vi "Confocal_0919_withZstep.vi"() -> ()   [LabVIEW 2017]
uses:
  <vilib>/Math Plots/2D Math Plots/XY Plot Matrix/XY Plot Matrix XCtrl/XY Plot Matrix.xctl
  Public/Documents/SIToolkit/LabVIEW/ExamplesXX_4_3_1_4/Spectroscopy Applications/GlobalCamOpen.vi
  Public/Documents/SIToolkit/LabVIEW/ExamplesXX_4_3_1_4/Spectroscopy Applications/GlobalInitializeFlag.vi
  Desktop/GlobalTimingMode-edit.vi
  Public/Documents/SIToolkit/LabVIEW/ExamplesXX_4_3_1_4/Spectroscopy Applications/GlobalFramesToStr.vi
  Public/Documents/SIToolkit/LabVIEW/ExamplesXX_4_3_1_4/Spectroscopy Applications/GlobalAcquireFocusFlag.vi
  Public/Documents/SIToolkit/LabVIEW/ExamplesXX_4_3_1_4/Spectroscopy Applications/GlobalExposure.vi
  <vilib>/Math Plots/2D Math Plots/XY Plot Matrix/XY Plot Matrix Datatype/XY Plot Matrix Datatype.lvclass
panel:
  out "Position 6":dbl[](array[numeric]) format="%.6f"
  out "Position 7":dbl[](array[numeric]) format="%.6f"
  out "Position 4":dbl[](array[numeric]) format="%.6f"
  in  "error PI Stage":errorcluster
  out "error out 2":errorcluster
  in  "Tab Control":T1(tab)
  in  "Focus/Acquire Mode":u32=1 min=1 max=5 step=1
  in  "Number of Frames to store":u32=1 min=1 step=1
  in  "Timing Mode":u32(ring)=1 items=["N/A", "Free Run/Timed", "Trigger First (PM only)", "Ext Sync/Strobed ", "Variable Exp (PM only)", "Flash Mode (PM only)"]
  out "Pixel Time":i32
  out "Bit Depth":i32
  out "ReadOut port":i32
  out "ADC Speed":i32
  in  "Set Experiment \nParameters, Initialize \nCamera/Controller":bool
  out "Read Temp.":dbl format="%.2f"
  in  "Set Temp.":dbl format="%.2f"
  in  "Exposure 2":dbl=0.2 format="%.2f"
  out "Controller Initialized":bool
  in  "error in":errorcluster
  out "error out":errorcluster
  in  "Power":dbl=10.0
  in  "Frequency":dbl=2810.0
  in  "Release Camera":bool
  out "Camera Opened":bool
  out "COM Error":bool
  in  "Serial Port":refnum<visa-resource-name>="COM3"
  in  "Number of Steps Left (must be even)":dbl=5.0 format="%#_13g"
  in  "OK Button 5":bool
  in  "Step Size (microns)":dbl[](array[numeric])=[0.01]
  out "XY Plot Matrix":refnum<class "XY Plot Matrix Datatype.lvclass">[](xcontrol)
  in  "Number of Steps Down":dbl=5.0 format="%#_13g"
  out "Position":dbl[](array[numeric]) format="%.6f"
  out "Position 3":dbl[](array[numeric]) format="%.6f"
  in  "stop 2":bool
  out "Position 2":dbl[](array[numeric]) format="%.6f"
  out "loop iteration":i32
  in  "Step Size (microns) Z":dbl[](array[numeric])=[0.01]
  out "Execution Time (ms)":u32
  in  "?":bool
  out "Position 5":dbl[](array[numeric]) format="%.6f"
  in  "Step Size (microns) Y":dbl[](array[numeric])=[0.01]
  in  "Step Size (microns) X":dbl[](array[numeric])=[0.01]
  out "Position 8":dbl[](array[numeric]) format="%.6f"
  in  "?":bool
  out "Acquire Graph":sgl[](graph)
  out "Collecting Data":bool
  in  "Full File Name for Acqure":path
  in  "OK Button":bool
  # "The following are read \nfrom camera after setting\nvalues to left.\n-1 value means item is not \nsupported by camera."
  # "Stage position on connection."
  # "Be sure to put in a full file name below before starting."
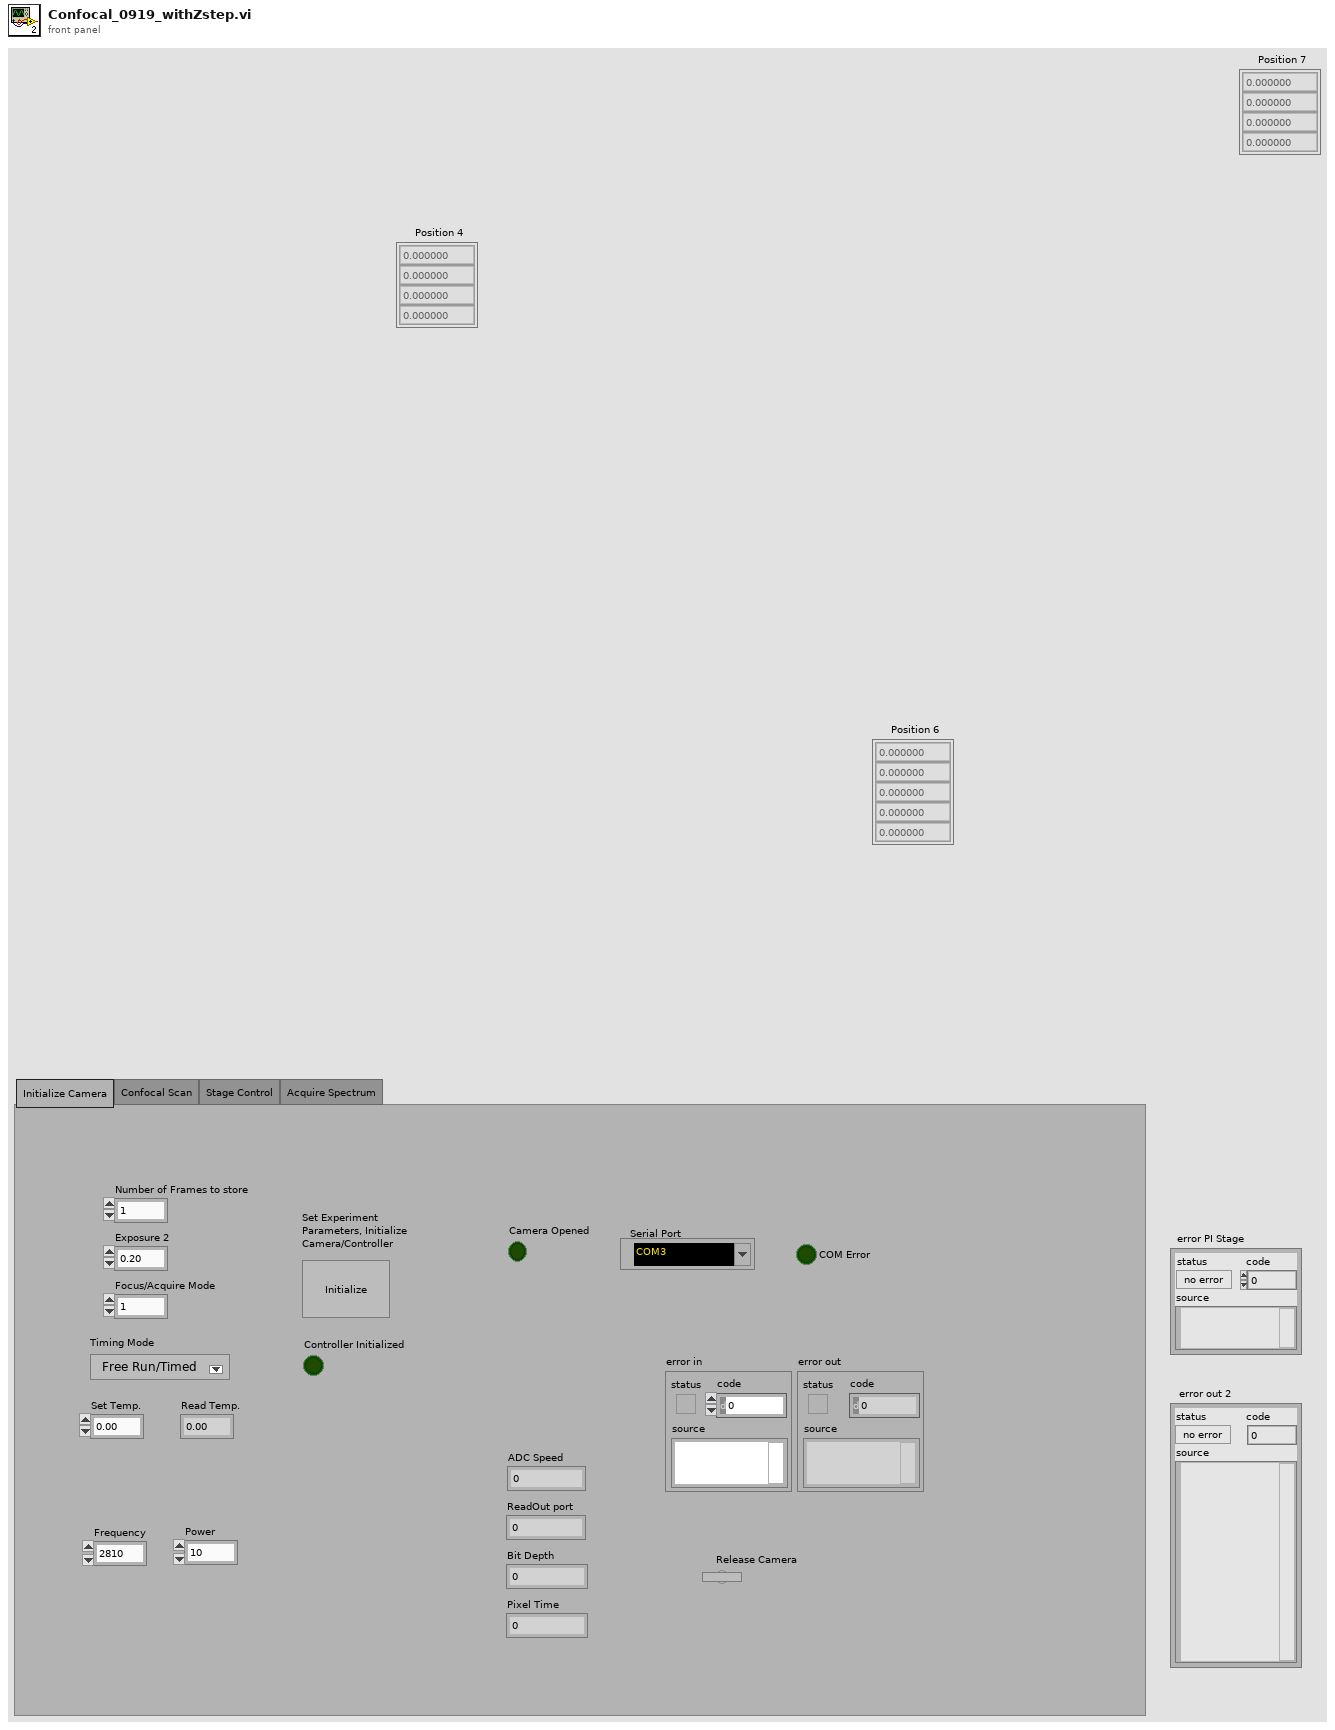
[diagram p1: front panel]
types:
  T1 = enum32{"Initialize Camera", "Confocal Scan", "Stage Control", "Acquire Spectrum"}
  T2 = cluster{"X start":u32, "X end":u32, "X Binning/Grouping":u32, "Y start":u32, "Y end":u32, "Y Binning/Grouping":u32}
  T3 = cluster{"Camera Handle":u32, "Pulser Handle":u32, "File Handle":u32, "Display Handle":u32, "Image Handle":u32}
  T4 = cluster{"Host address/name":string, "Port":i32, "Board":i32, "TCP/IP Search?":bool}
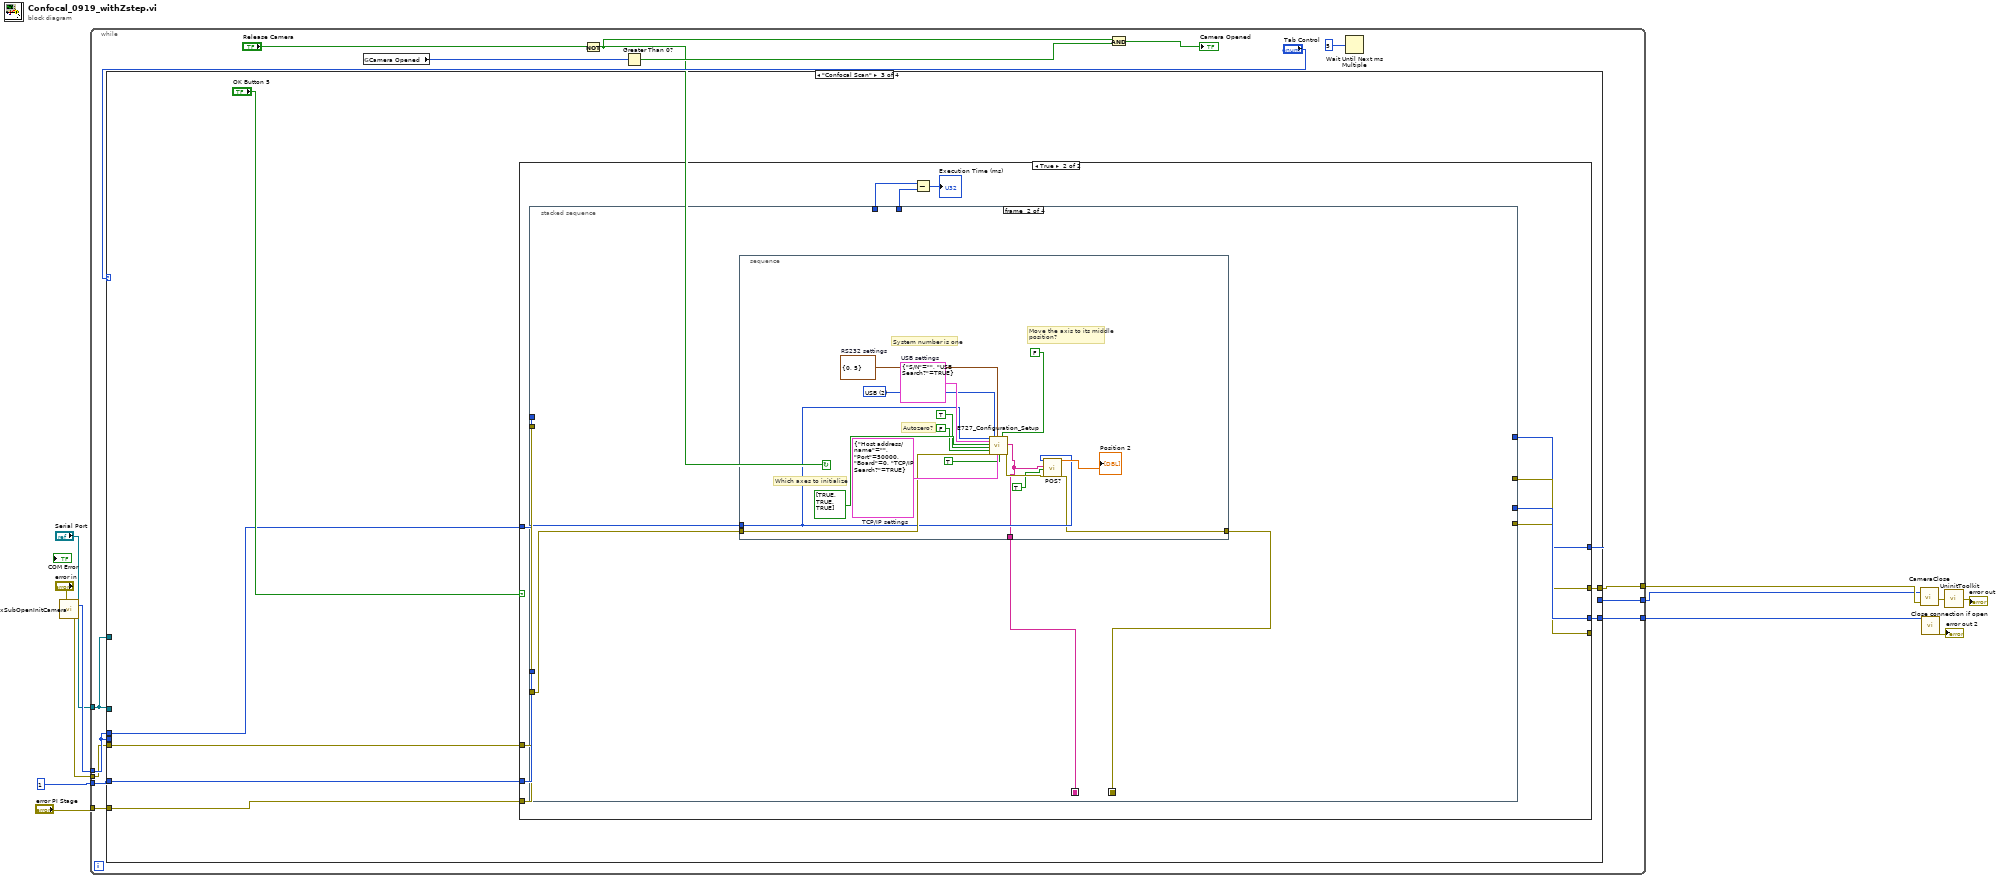
[diagram p0: block diagram]
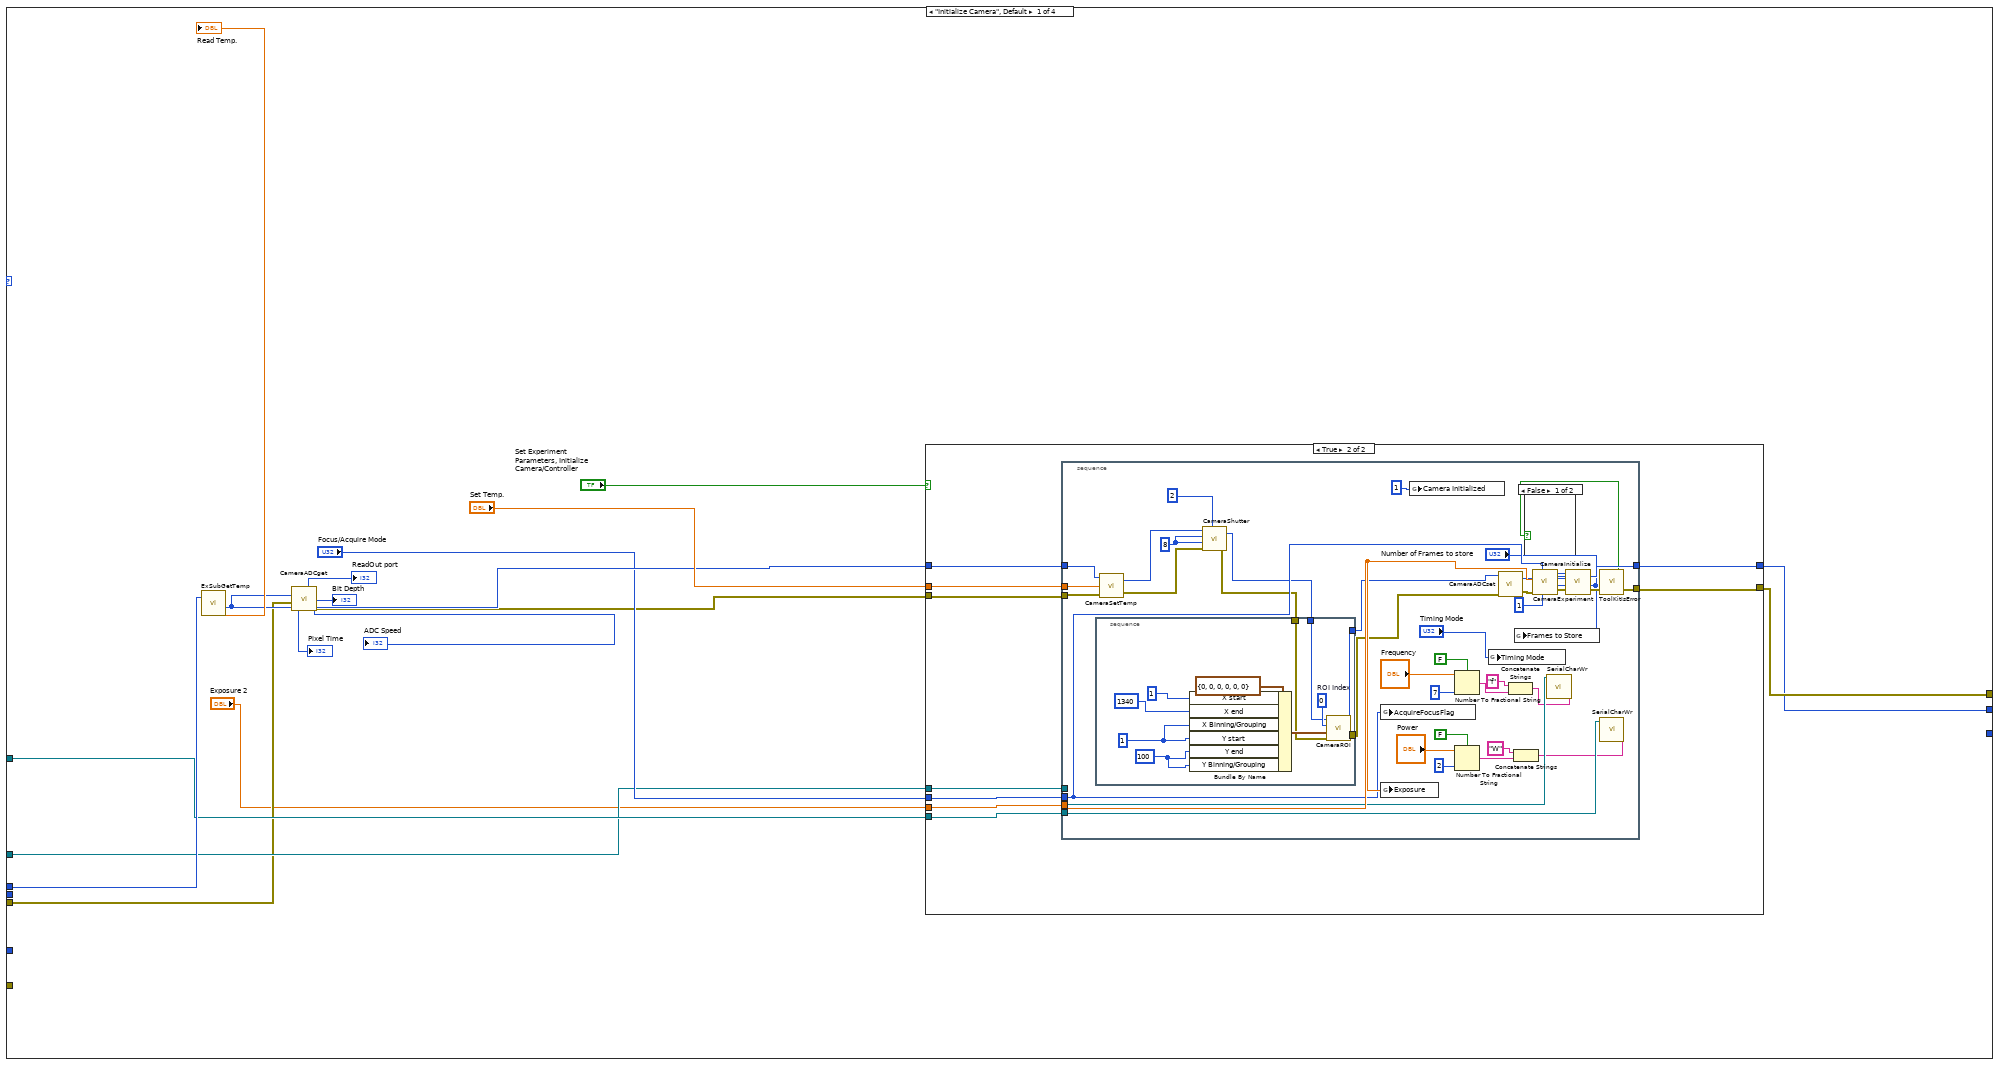
[diagram p2: hidden frame]
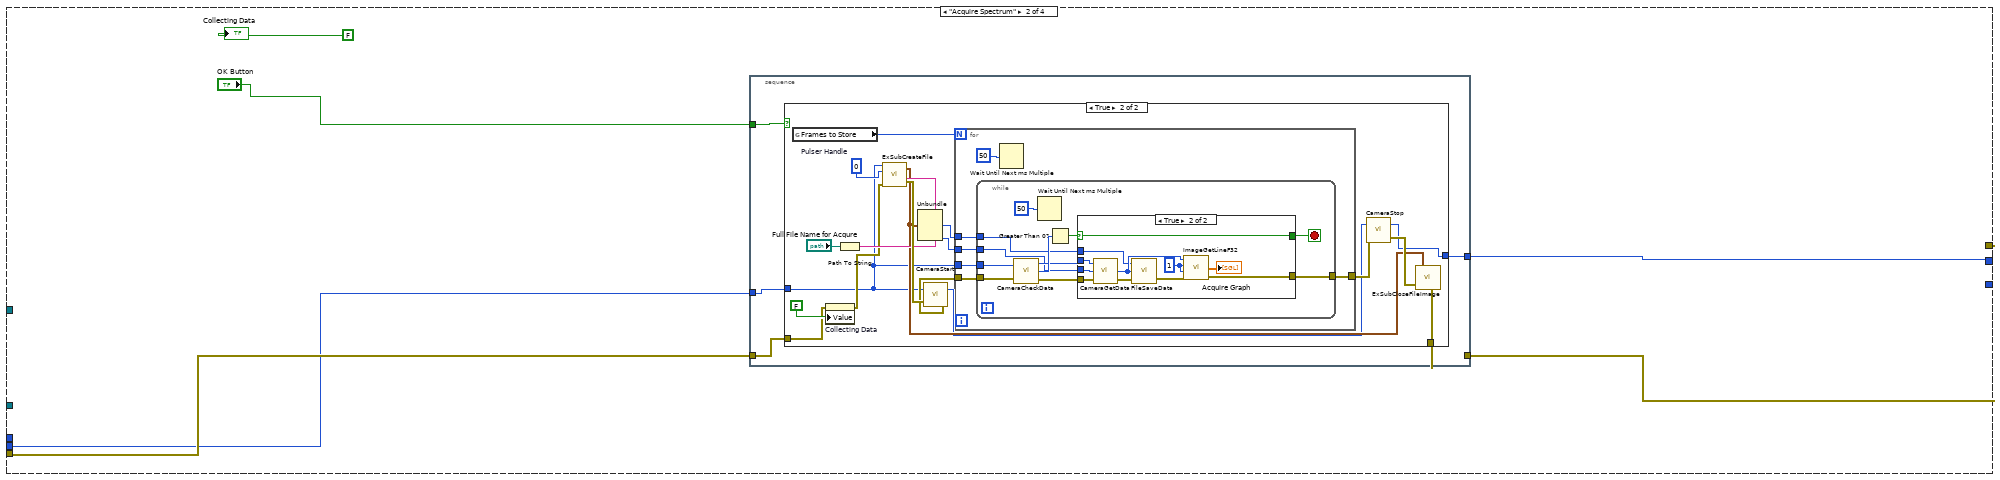
[diagram p5: hidden frame]
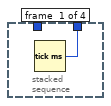
[diagram p9: hidden frame]
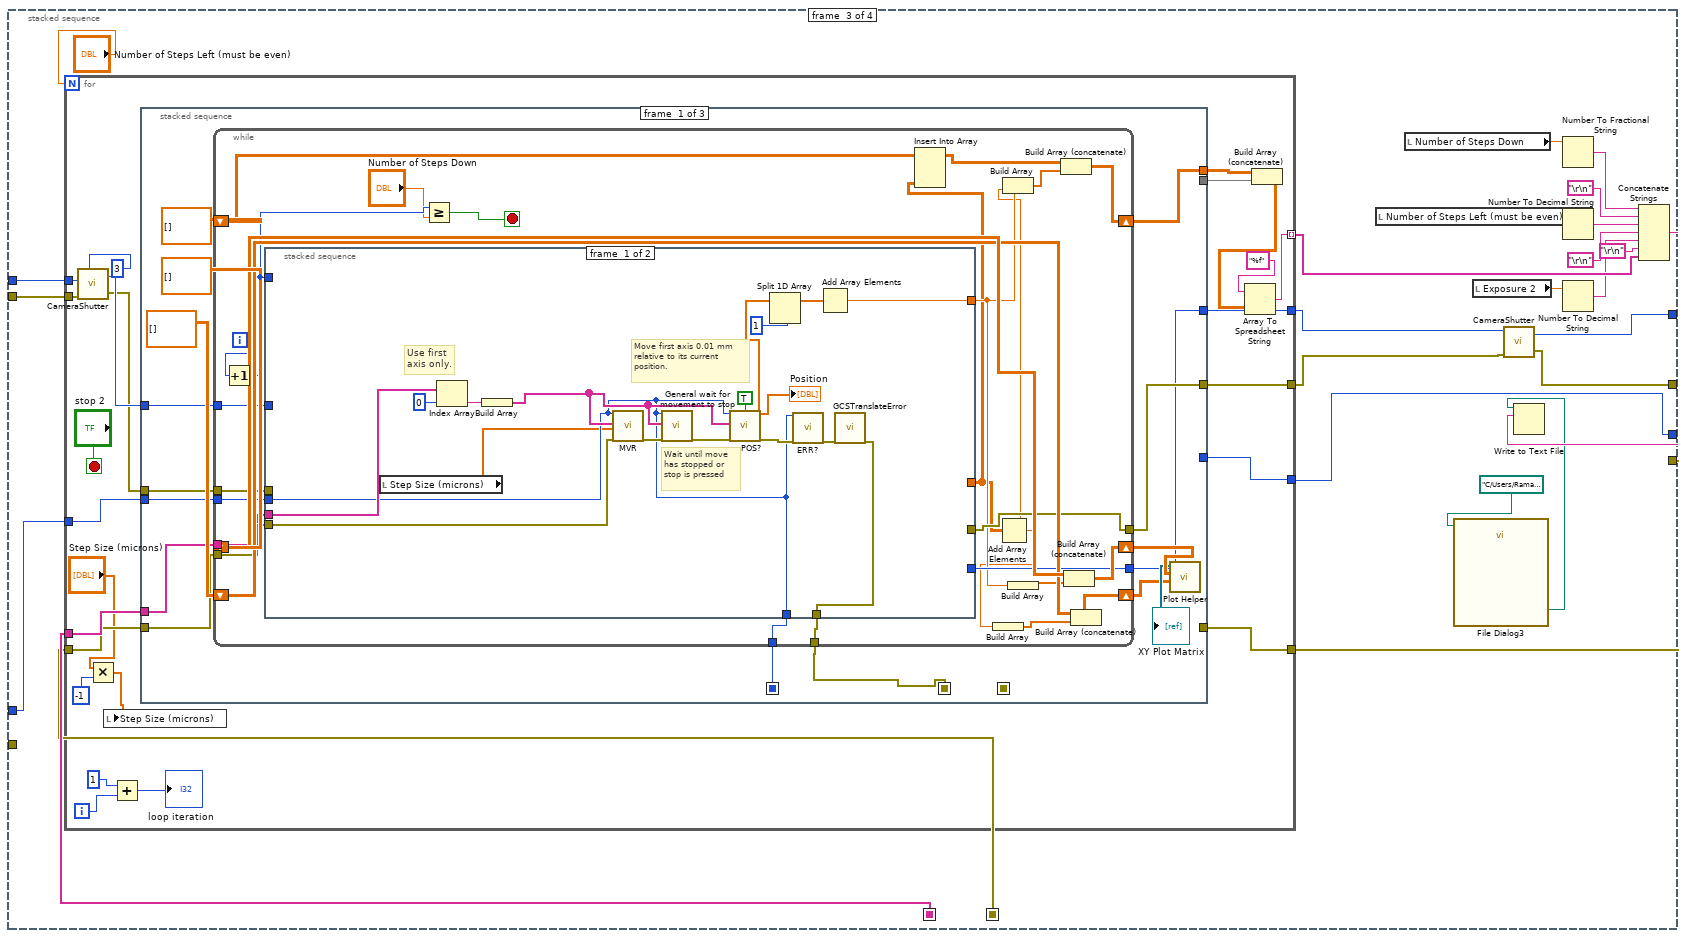
[diagram p10: hidden frame]
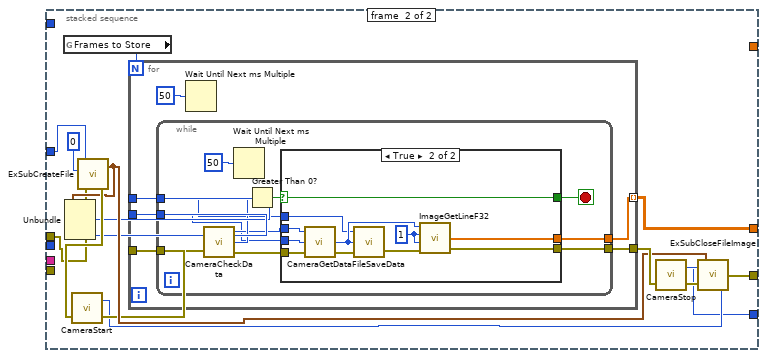
[diagram p11: hidden frame]
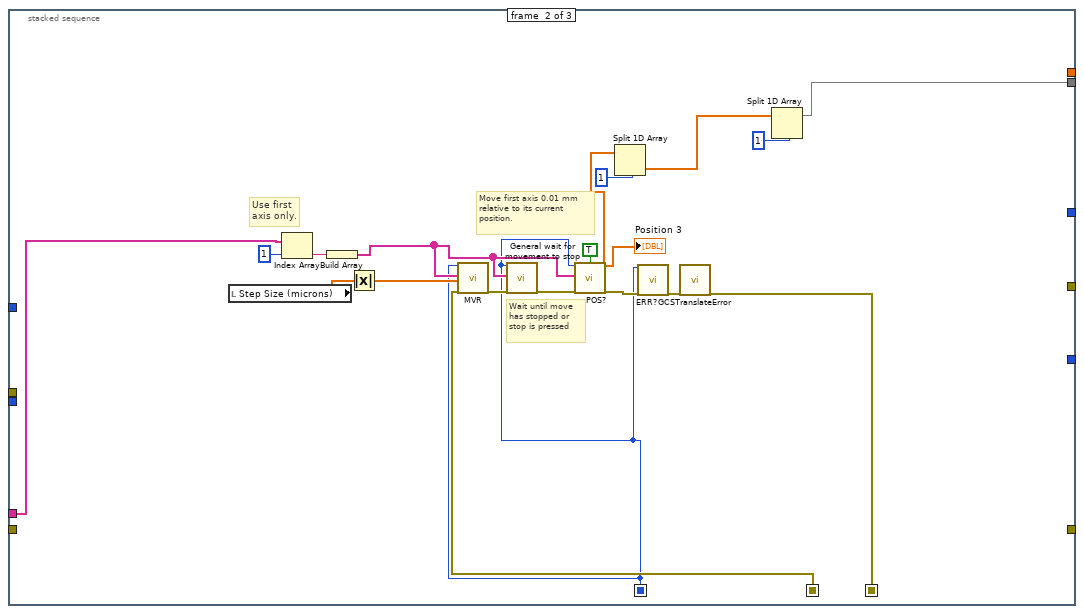
[diagram p13: hidden frame]
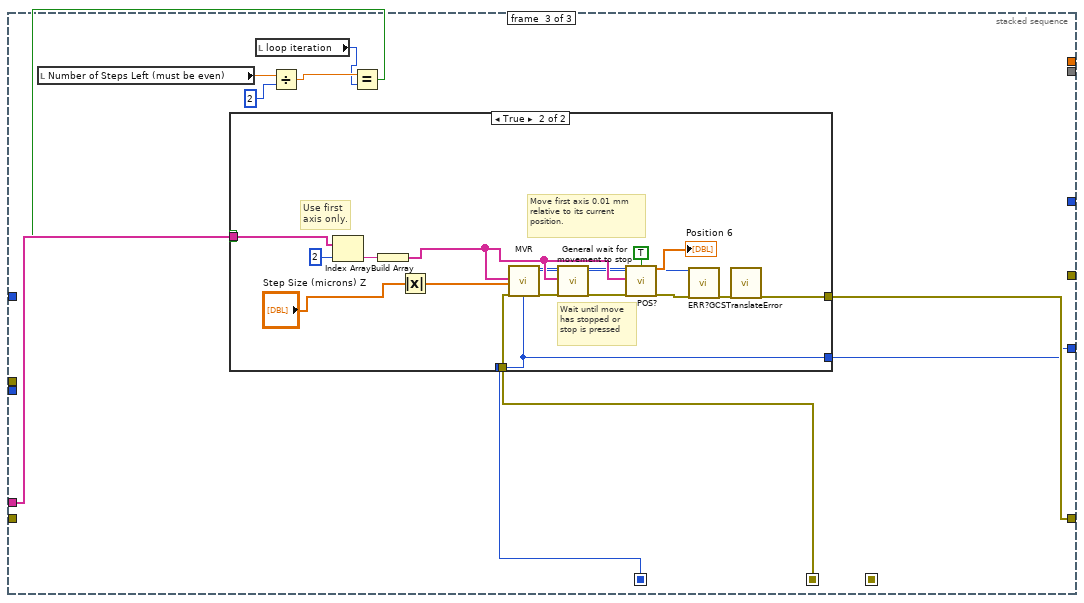
[diagram p14: hidden frame]
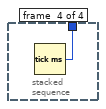
[diagram p16: hidden frame]
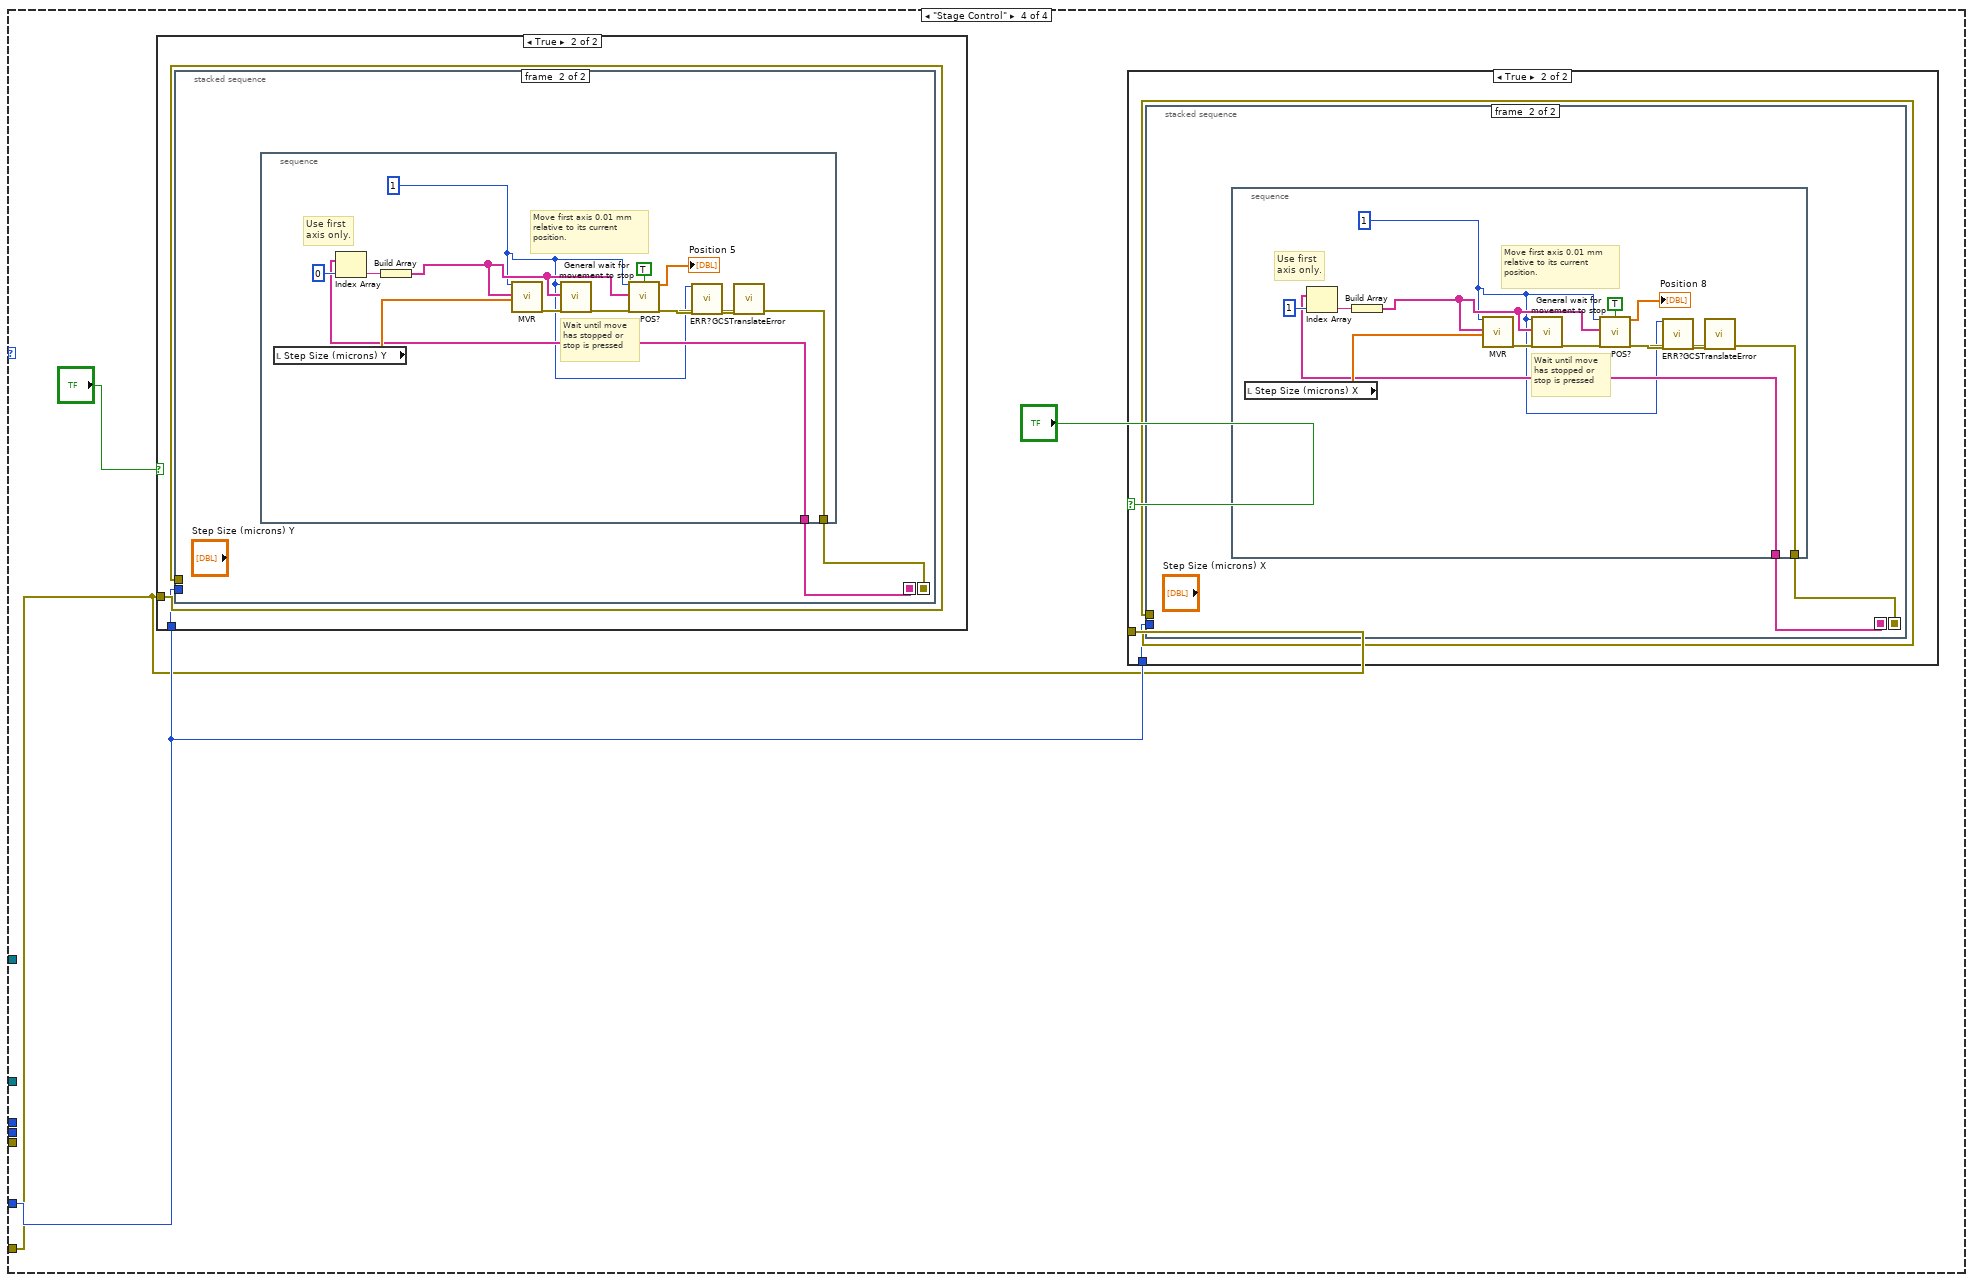
[diagram p17: hidden frame]
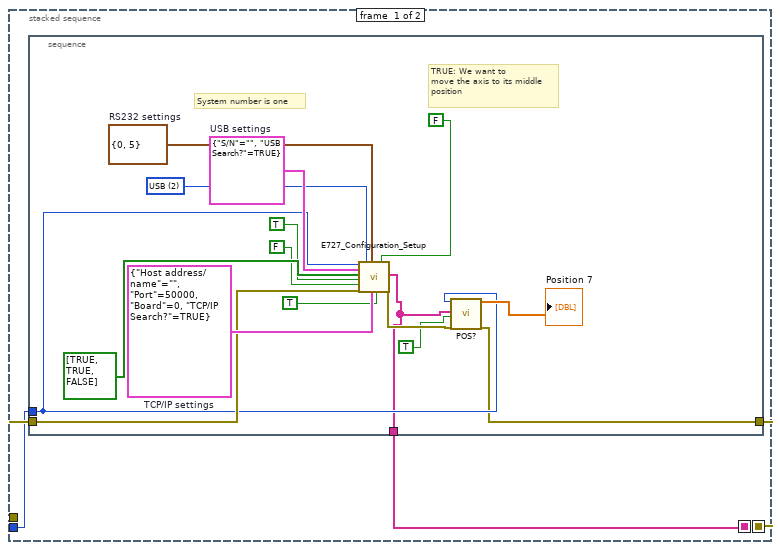
[diagram p19: hidden frame]
diagram:
  n1 = call "ExSubOpenInitCamera.vi"("error in (no error)"="error in") -> ("Camera Handle"=w11:u32, "error out"=w9:errorcluster)
  n2 = while {
    tunnel: w11 -> [w20]
    tunnel: "Serial Port" -> [w21]
    tunnel: w9 -> [w19]
    tunnel: [w18] -> w8
    tunnel: [w16] -> w5
    tunnel: "error PI Stage" -> [w15]
    tunnel: 1 -> [w13]
    tunnel: [w14] -> w1
    stop <- w17 continue-if-true
    n3 = case shown="\"Confocal Scan\"" "Tab Control" {
      tunnel: w20 -> [w36 _ w169 _]
      tunnel: w21 -> [w35 _ _ _]
      tunnel: w21 -> [w34 _ _ _]
      tunnel: w20 -> [_ w111 _ _]
      tunnel: w19 -> [w33 w112 w170 _]
      tunnel: [w28 w108 w171 _] -> w16
      tunnel: [w30 w109 w172 _] -> w18
      tunnel: w15 -> [_ _ w174 w409]
      tunnel: w13 -> [_ _ w176 w410]
      tunnel: [_ _ w175 _] -> w14
      frame "Initialize Camera", Default {
        n4 = call "ExSubGetTemp.vi"("Camera Handle"=w36) -> ("Camera Handle"=w41:u32, "Temperature Real"=→"Read Temp.":dbl)  [unwired: 1 in, 1 out]
        n5 = call <userlib>:"CameraADCget.vi"("Camera handle"=w41, "error in (no error)"=w33) -> ("Bit Depth"=→"Bit Depth":i32, "Pixel Time"=→"Pixel Time":i32, "Readout Port"=→"ReadOut port":i32, "ADC Speed"=→"ADC Speed":i32, "error out"=w32:errorcluster)  [unwired: 3 out]
        n6 = case shown="True" "Set Experiment \nParameters, Initialize \nCamera/Controller" {
          tunnel: "Exposure 2" -> [_ w55]
          tunnel: "Set Temp." -> [_ w56]
          tunnel: w41 -> [w48 w57]
          tunnel: [w48 w54] -> w28
          tunnel: "Focus/Acquire Mode" -> [_ w53]
          tunnel: w35 -> [_ w52]
          tunnel: w34 -> [_ w51]
          tunnel: w32 -> [w47 w50]
          tunnel: [w47 w49] -> w30
          frame False {
          }
          frame True {
            n7 = stacked-sequence {
              tunnel: w57 -> [w96]
              tunnel: w56 -> [w95]
              tunnel: w55 -> [w94]
              tunnel: [w93] -> w54
              tunnel: w53 -> [w92]
              tunnel: w52 -> [w91]
              tunnel: w51 -> [w90]
              tunnel: w50 -> [w89]
              tunnel: [w88] -> w49
              frame #0 {
                w58 = 8
                n8 = call <userlib>:"CameraSetTemp.vi"("error in (no error)"=w89, "Temperature"=w95, "Camera Handle"=w96) -> ("error out"=w61:errorcluster, "Camera Handle"=w63:u32)
                n9 = call <userlib>:"CameraShutter.vi"("Camera Handle"=w63, "Shutter Comp Time: Pre Open"=w58, "Shutter Comp Time: Post Open"=w58, "error in"=w61, "Shutter State"=2) -> ("Camera Handle"=w62:u32, "error out"=w60:errorcluster)
                n10 = stacked-sequence {
                  tunnel: [w104] -> w65
                  tunnel: w62 -> [w101]
                  tunnel: w60 -> [w100]
                  tunnel: [w99] -> w64
                  frame #0 {
                    w103 = 100
                    w97 = 1
                    w106 = u32 0  # ROI Index
                    n11 = Bundle By Name(cluster=T2 {"X start"=0, "X end"=0, "X Binning/Grouping"=0, "Y start"=0, "Y end"=0, "Y Binning/Grouping"=0} ("ROI Params"), "X start"=1, "X end"=1340, "X Binning/Grouping"=w97, "Y start"=w97, "Y end"=w103, "Y Binning/Grouping"=w103) -> (w107:T2)
                    n12 = call <userlib>:"CameraROI.vi"("error in"=w100, "ROI Params"=w107, "ROI Index"=w106, "Camera Handle"=w101) -> ("error out"=w99:errorcluster, "Camera Handle"=w104:u32)
                  }
                }
                n13 = global write "GlobalAcquireFocusFlag.vi" "AcquireFocusFlag"(w92) -> ()
                n14 = global write "GlobalExposure.vi" "Exposure"(w94) -> ()
                n15 = global write "GlobalInitializeFlag.vi" "Camera Initialized"(1) -> ()
                n16 = Number To Fractional String(use system decimal point (T)=FALSE, number="Frequency", precision (6)=7) -> (F-format string=w67:string)  [unwired: 1 in]
                n17 = Number To Fractional String(use system decimal point (T)=FALSE, number="Power", precision (6)=2) -> (F-format string=w75:string)  [unwired: 1 in]
                n18 = global write "GlobalTimingMode-edit.vi" "Timing Mode"("Timing Mode") -> ()
                n19 = call <userlib>:"CameraADCset.vi"("error in (no error)"=w64, "Camera Handle"=w65) -> ("error out"=w84:errorcluster, "Camera Handle"=w83:u32)  [unwired: 4 in]
                n20 = Concatenate Strings("f", w67) -> (w73:string)
                n21 = Concatenate Strings("W", w75) -> (w76:string)
                n22 = global write "GlobalFramesToStr.vi" "Frames to Store"("Number of Frames to store") -> ()
                n23 = call <userlib>:"CameraExperiment.vi"("Number of Accumulations"=1, "Acquire / Focus Flag"=w92, "error in"=w84, "Number of Images"="Number of Frames to store", "Exposure (sec)"=w94, "Camera Handle"=w83) -> ("error out"=w82:errorcluster, "Camera Handle"=w81:u32)
                n24 = call "SerialCharWr.vi"("VISA resource name"=w90, "write buffer"=w73) -> ()  [unwired: 6 in, 3 out]
                n25 = call <userlib>:"CameraInitialize.vi"("error in"=w82, "Camera Handle"=w81) -> ("error out"=w79:errorcluster, "Camera Handle"=w93:u32)
                n26 = call <userlib>:"ToolKitIsError.vi"("error in"=w79) -> ("error out"=w88:errorcluster, "Error Flag"=w80:bool)  [unwired: 1 in]
                n27 = case shown="False" w80 {
                  frame False {
                  }
                  frame True {
                  }
                }
                n28 = call "SerialCharWr.vi"("VISA resource name"=w91, "write buffer"=w76) -> ()  [unwired: 6 in, 3 out]
              }
            }
          }
        }
        n29 = global read "GlobalInitializeFlag.vi" "Camera Initialized"() -> (w44:u32)
        n30 = Greater Than 0?(x=w44) -> (x > 0?=→"Controller Initialized":bool)
      }
      frame "Acquire Spectrum" {
        n31 = stacked-sequence {
          tunnel: [w115] -> w109
          tunnel: [w116] -> w108
          tunnel: w112 -> [w118]
          tunnel: "OK Button" -> [w117]
          tunnel: w111 -> [w114]
          frame #0 {
            n32 = case shown="True" w117 {
              tunnel: [w119 w131] -> w116
              tunnel: [w120 w123] -> w115
              tunnel: w118 -> [w120 w122]
              tunnel: w114 -> [w119 w121]
              frame False {
              }
              frame True {
                w125 = u32 0  # Pulser Handle
                n33 = global read "GlobalFramesToStr.vi" "Frames to Store"() -> (w134:u32)
                n34 = property on="Collecting Data" class="Bool (strict)"(error in=w122, "Value"=FALSE) -> (error out=w133:errorcluster)  [unwired: 1 in, 1 out]
                n35 = Path To String(path="Full File Name for Acqure") -> (string=w136:string)
                n36 = call "ExSubCreateFile.vi"("error in (no error)"=w133, "File and Display Name"=w136, "Pulser Handle"=w125, "Camera Handle"=w121) -> ("error out"=w138:errorcluster, "Handles Out"=w129:T3)
                n37 = Unbundle(w129) -> ("File Handle"=w124:u32, "Image Handle"=w127:u32)  [unwired: 3 out]
                n38 = call <userlib>:"CameraStart.vi"("error in"=w138, "Camera Handle"=w121) -> ("error out"=w128:errorcluster, "Camera Handle"=w126:u32)
                n39 = for {
                  N: w134 -> [_]
                  tunnel: w121 -> [w143]
                  tunnel: w128 -> [w142]
                  tunnel: [w141] -> w130
                  tunnel: w124 -> [w140]
                  tunnel: w127 -> [w139]
                  n40 = while {
                    tunnel: [w150] -> w141
                    tunnel: w143 -> [w148]
                    tunnel: w142 -> [w147]
                    tunnel: w140 -> [w146]
                    tunnel: w139 -> [w145]
                    stop <- w151 stop-if-true
                    n41 = call <userlib>:"CameraCheckData.vi"("Camera Handle"=w148, "error in"=w147) -> ("Camera Handle"=w153:u32, "Number Of Frames Available"=w155:i32, "error out"=w152:errorcluster)
                    n42 = Wait Until Next ms Multiple(millisecond multiple=u32 50) -> ()  [unwired: 1 out]
                    n43 = Greater Than 0?(x=w155) -> (x > 0?=w154:bool)
                    n44 = case shown="True" w154 {
                      selector: w154 -> [w156 w166]
                      tunnel: w153 -> [_ w168]
                      tunnel: w152 -> [w157 w167]
                      tunnel: [w156 w166] -> w151
                      tunnel: [w157 w161] -> w150
                      tunnel: w146 -> [_ w159]
                      tunnel: w145 -> [_ w158]
                      frame False {
                      }
                      frame True {
                        w162 = 1
                        n45 = call <userlib>:"CameraGetData.vi"("error in"=w167, "Image/Data Handle"=w158, "Camera Handle"=w168) -> ("error out"=w165:errorcluster, "Image/Data Handle"=w163:u32)  [unwired: 1 out]
                        n46 = call <userlib>:"FileSaveData.vi"("error in"=w165, "Image Handle"=w163, "File Handle"=w159) -> ("error out"=w164:errorcluster)  [unwired: 1 out]
                        n47 = call <userlib>:"ImageGetLineF32.vi"("error in"=w164, "Z Position"=w162, "Y Position"=w162, "Data Handle"=w163) -> ("error out"=w161:errorcluster, "Array F32"=→"Acquire Graph":sgl[])  [unwired: 1 out]
                      }
                    }
                  }
                  n48 = Wait Until Next ms Multiple(millisecond multiple=u32 50) -> ()  [unwired: 1 out]
                }
                n49 = call <userlib>:"CameraStop.vi"("error in"=w130, "Camera Handle"=w126) -> ("error out"=w135:errorcluster, "Camera Handle"=w131:u32)
                n50 = call "ExSubCloseFileImage.vi"("error in (no error)"=w135, "Handles In"=w129) -> ("error out"=w123:errorcluster)
              }
            }
          }
        }
        "Collecting Data" <- FALSE
      }
      frame "Confocal Scan" {
        n51 = case shown="True" "OK Button 5" {
          tunnel: w176 -> [_ w187]
          tunnel: [_ w186] -> w175
          tunnel: [_ w185] -> _
          tunnel: w174 -> [_ w184]
          tunnel: [_ w183] -> w172
          tunnel: [_ w182] -> w171
          tunnel: w170 -> [_ w181]
          tunnel: w169 -> [_ w180]
          frame False {
          }
          frame True {
            n52 = stacked-sequence {
              seq-local: [_ w190 _ _] -> [_ _ w230 _]
              seq-local: [_ w189 _ _] -> [_ _ w229 _]
              tunnel: w187 -> [_ w191 w233 _]
              tunnel: [_ _ w232 _] -> w186
              tunnel: [_ _ w231 _] -> w185
              tunnel: w184 -> [_ w192 _ _]
              tunnel: [_ _ w222 _] -> w183
              tunnel: [_ _ w224 _] -> w182
              tunnel: w181 -> [_ _ w221 _]
              tunnel: w180 -> [_ _ w220 _]
              tunnel: [w188 _ _ _] -> w179
              tunnel: [_ _ _ w408] -> w178
              frame #0 {
                n53 = Tick Count (ms)() -> (millisecond timer value=w188:u32)
              }
              frame #1 {
                # "Which axes to initialize"
                n54 = stacked-sequence {
                  tunnel: w192 -> [w196]
                  tunnel: w191 -> [w195]
                  tunnel: [w194] -> w189
                  tunnel: [w193] -> w190
                  frame #0 {
                    w208 = cluster{"S/N":string, "USB Search?":bool} {"S/N"="", "USB Search?"=TRUE}  # USB settings
                    w204 = u16 2 items=["RS232", "TCP/IP", "USB"] ("Interface")
                    w203 = cluster{"Portnumber":i32, "Baudrate":u16} {"Portnumber"=0, "Baudrate"=5}  # RS232 settings
                    w202 = T4 {"Host address/name"="", "Port"=50000, "Board"=0, "TCP/IP Search?"=TRUE}  # TCP/IP settings
                    # "Autozero?"
                    # "Move the axis to its middle\nposition?"
                    # "System number is one"
                    n55 = call "E727_Configuration_Setup.vi"("System no."=w195, "USB settings"=w208, "Are stages connected?"=bool[] [TRUE, TRUE, TRUE], "Change servo status to ON?"=TRUE ("Use dialog to define\nconnected stages?"), "Perform autozero?"=FALSE ("Use dialog to define\nconnected stages?"), "error in"=w196, "Interface"=w204, "RS232 settings"=w203, "TCP/IP settings"=w202, "Stop wave generator\noutput (if any)"=TRUE ("All axes?"), "Move to middle?"=FALSE) -> ("All conn. axes"=w193:string[], "error out"=w198:errorcluster)  [unwired: 3 in, 4 out]
                    n56 = call "POS?.vi"("System no."=w195, "Axes to query"=w193, "All axes?"=TRUE, "error in"=w198) -> ("Position"=→"Position 2":dbl[], "error out"=w194:errorcluster)  [unwired: 1 in, 13 out]
                  }
                }
              }
              frame #2 {
                n57 = for {
                  N: "Number of Steps Left (must be even)" -> [_]
                  tunnel: w233 -> [w254]
                  tunnel: [w248] -> w219 mode=indexing
                  tunnel: [w256] -> w231
                  tunnel: w230 -> [w255]
                  tunnel: w229 -> [w253]
                  tunnel: [w252] -> w232
                  tunnel: [w244] -> w223
                  tunnel: [w243] -> w225
                  tunnel: w221 -> [w239]
                  tunnel: w220 -> [w238]
                  i -> [w236]
                  stop <- "stop 2" stop-if-true
                  n58 = call <userlib>:"CameraShutter.vi"("Shutter Comp Time: Pre Open"=w238, "error in"=w239, "Shutter State"=3) -> ("Camera Handle"=w241:u32, "error out"=w240:errorcluster)  [unwired: 2 in]
                  n59 = Multiply(x="Step Size (microns)", y=-1) -> (x*y=w249:dbl[])
                  n60 = local write "Step Size (microns)"(w249) -> ()
                  n61 = Add(x=1, y=w236) -> (x+y=→"loop iteration":i32)
                  n62 = stacked-sequence {
                    seq-local: [w264 _ _] -> [_ w362 w389]
                    seq-local: [w258 _ _] -> [_ w364 w387]
                    seq-local: [_ w363 _] -> [_ _ _]
                    tunnel: [_ _ w388] -> w256
                    tunnel: w255 -> [w267 w370 w390]
                    tunnel: w254 -> [w265 _ _]
                    tunnel: w253 -> [w266 _ _]
                    tunnel: [_ _ w386] -> w252
                    tunnel: [w263 _ _] -> w246
                    tunnel: [_ w365 _] -> w237
                    tunnel: [w262 _ _] -> w244
                    tunnel: [w261 _ _] -> w243
                    tunnel: w241 -> [w260 _ _]
                    tunnel: w240 -> [w259 _ _]
                    frame #0 {
                      n63 = while {
                        shift-right: [w293] -> w271
                        shift-left: dbl[][] [] -> [w298]
                        shift-right: [w296] -> w268
                        shift-left: dbl[][] [] -> [w297]
                        shift-right: [w274] -> w263
                        shift-left: dbl[][] [] -> [w277]
                        tunnel: w266 -> [w295]
                        tunnel: w267 -> [w294]
                        tunnel: w265 -> [w289]
                        tunnel: [w288] -> w258
                        tunnel: [w287] -> w264
                        tunnel: [w284] -> w262
                        tunnel: [w283] -> w261
                        tunnel: w260 -> [w282]
                        tunnel: w259 -> [w281]
                        i -> [w290]
                        stop <- w292 stop-if-true
                        n64 = Increment(x=w290) -> (x+1=w286:i32)
                        n65 = stacked-sequence {
                          tunnel: w295 -> [w316 _]
                          tunnel: [w309 _] -> w288
                          tunnel: w294 -> [w307 _]
                          tunnel: w286 -> [_ _]
                          tunnel: [w302 _] -> w280
                          tunnel: w289 -> [w301 _]
                          tunnel: [w301 _] -> w287
                          tunnel: [_ w321] -> w278
                          tunnel: [_ w320] -> w284
                          tunnel: [_ w319] -> w283
                          tunnel: w282 -> [_ w318]
                          tunnel: w281 -> [_ w317]
                          frame #0 {
                            # "Use first\naxis only."
                            # "Wait until move\nhas stopped or\nstop is pressed"
                            # "Move first axis 0.01 mm\nrelative to its current\nposition."
                            n66 = local read "Step Size (microns)"() -> (w300:dbl[])
                            n67 = Index Array(array=w307, index=0) -> (element=w310:string)
                            n68 = Build Array(w310) -> (w306:string[])
                            n69 = call "MVR.vi"("System no."=w301, "Axes to move"=w306, "Position values"=w300, "error in"=w316) -> ("error out"=w314:errorcluster)  [unwired: 1 in, 14 out]
                            n70 = call "General wait for movement to stop.vi"("System no."=w301, "Axes to wait for"=w306, "error in"=w314) -> ("error out"=w308:errorcluster)  [unwired: 5 in, 11 out]
                            n71 = call "POS?.vi"("System no."=w301, "Axes to query"=w306, "All axes?"=TRUE, "error in"=w308) -> ("Position"=w305:dbl[], "error out"=w313:errorcluster)  [unwired: 1 in, 13 out]
                            "Position" <- w305
                            n72 = Split 1D Array(array=w305, index=1) -> (first subarray=w303:dbl[])  [unwired: 1 out]
                            n73 = call "ERR?.vi"("System no."=w301, "error in"=w313) -> ("error out"=w312:errorcluster)  [unwired: 17 out]
                            n74 = Add Array Elements(numeric array=w303) -> (sum=w302:dbl)
                            n75 = call "GCSTranslateError.vi"("error in"=w312) -> ("error out"=w309:errorcluster)  [unwired: 18 out]
                          }
                          frame #1 {
                            n76 = global read "GlobalFramesToStr.vi" "Frames to Store"() -> (w329:u32)
                            n77 = call "ExSubCreateFile.vi"("error in (no error)"=w317, "Pulser Handle"=u32 0, "Camera Handle"=w318) -> ("error out"=w331:errorcluster, "Handles Out"=w327:T3)  [unwired: 1 in]
                            n78 = Unbundle(w327) -> ("File Handle"=w322:u32, "Image Handle"=w325:u32)  [unwired: 3 out]
                            n79 = call <userlib>:"CameraStart.vi"("error in"=w331) -> ("error out"=w326:errorcluster, "Camera Handle"=w324:u32)  [unwired: 1 in]
                            n80 = for {
                              N: w329 -> [_]
                              tunnel: w326 -> [w336]
                              tunnel: [w335] -> w328
                              tunnel: w322 -> [w334]
                              tunnel: w325 -> [w333]
                              tunnel: [w332] -> w321 mode=indexing
                              n81 = while {
                                tunnel: [w343] -> w335
                                tunnel: w336 -> [w341]
                                tunnel: w334 -> [w340]
                                tunnel: w333 -> [w339]
                                tunnel: [w338] -> w332
                                stop <- w344 stop-if-true
                                n82 = call <userlib>:"CameraCheckData.vi"("error in"=w341) -> ("Camera Handle"=w346:u32, "Number Of Frames Available"=w348:i32, "error out"=w345:errorcluster)  [unwired: 1 in]
                                n83 = Wait Until Next ms Multiple(millisecond multiple=u32 50) -> ()  [unwired: 1 out]
                                n84 = Greater Than 0?(x=w348) -> (x > 0?=w347:bool)
                                n85 = case shown="True" w347 {
                                selector: w347 -> [w349 w359]
                                tunnel: w346 -> [_ w361]
                                tunnel: w345 -> [w350 w360]
                                tunnel: [w349 w359] -> w344
                                tunnel: [w350 w354] -> w343
                                tunnel: w340 -> [_ w353]
                                tunnel: w339 -> [_ w352]
                                tunnel: [_ w351] -> w338
                                frame False {
                                }
                                frame True {
                                w355 = 1
                                n86 = call <userlib>:"CameraGetData.vi"("error in"=w360, "Image/Data Handle"=w352, "Camera Handle"=w361) -> ("error out"=w358:errorcluster, "Image/Data Handle"=w356:u32)  [unwired: 1 out]
                                n87 = call <userlib>:"FileSaveData.vi"("error in"=w358, "Image Handle"=w356, "File Handle"=w353) -> ("error out"=w357:errorcluster)  [unwired: 1 out]
                                n88 = call <userlib>:"ImageGetLineF32.vi"("error in"=w357, "Z Position"=w355, "Y Position"=w355, "Data Handle"=w356) -> ("error out"=w354:errorcluster, "Array F32"=w351:sgl[])  [unwired: 1 out]
                                }
                                }
                              }
                              n89 = Wait Until Next ms Multiple(millisecond multiple=u32 50) -> ()  [unwired: 1 out]
                            }
                            n90 = call <userlib>:"CameraStop.vi"("error in"=w328, "Camera Handle"=w324) -> ("error out"=w330:errorcluster, "Camera Handle"=w319:u32)
                            n91 = call "ExSubCloseFileImage.vi"("error in (no error)"=w330, "Handles In"=w327) -> ("error out"=w320:errorcluster)
                          }
                        }
                        n92 = Greater Or Equal?(x=w286, y="Number of Steps Down") -> (x >= y?=w292:bool)
                        n93 = Insert Into Array(array=w277, new element=w278) -> (w275:dbl[][])  [unwired: 2 in]
                        n94 = Add Array Elements(numeric array=w278) -> (sum=w279:sgl)
                        n95 = Build Array(w279) -> (w299:sgl[])
                        n96 = Build Array(w280, w279) -> (w276:dbl[])
                        n97 = Build Array(w280) -> (w291:dbl[])
                        n98 = Build Array (concatenate)(w275, w276) -> (w274:dbl[][])
                        n99 = Build Array (concatenate)(w298, w291) -> (w293:dbl[][])
                        n100 = Build Array (concatenate)(w297, w299) -> (w296:dbl[][])
                      }
                      n101 = call <vilib>:"Plot Helper.vi"("y matrix"=w268, "x matrix"=w271) -> ("2D Plotmatrix Class Obj Array out"=→"XY Plot Matrix":refnum<class "XY Plot Matrix Datatype.lvclass">[])  [unwired: 2 in, 7 out]
                    }
                    frame #1 {
                      # "Use first\naxis only."
                      # "Wait until move\nhas stopped or\nstop is pressed"
                      # "Move first axis 0.01 mm\nrelative to its current\nposition."
                      n102 = local read "Step Size (microns)"() -> (w367:dbl[])
                      n103 = Index Array(array=w370, index=1) -> (element=w375:string)
                      n104 = Build Array(w375) -> (w373:string[])
                      n105 = Absolute Value(x=w367) -> (abs(x)=w366:dbl[])
                      n106 = call "MVR.vi"("System no."=w362, "Axes to move"=w373, "Position values"=w366, "error in"=w364) -> ("error out"=w379:errorcluster)  [unwired: 1 in, 14 out]
                      n107 = call "General wait for movement to stop.vi"("System no."=w362, "Axes to wait for"=w373, "error in"=w379) -> ("error out"=w374:errorcluster)  [unwired: 5 in, 11 out]
                      n108 = call "POS?.vi"("System no."=w362, "Axes to query"=w373, "All axes?"=TRUE, "error in"=w374) -> ("Position"=w372:dbl[], "error out"=w378:errorcluster)  [unwired: 1 in, 13 out]
                      "Position 3" <- w372
                      n109 = Split 1D Array(array=w372, index=1) -> (second subarray=w368:dbl[])  [unwired: 1 out]
                      n110 = call "ERR?.vi"("System no."=w362, "error in"=w378) -> ("error out"=w377:errorcluster)  [unwired: 17 out]
                      n111 = call "GCSTranslateError.vi"("error in"=w377) -> ("error out"=w363:errorcluster)  [unwired: 18 out]
                      n112 = Split 1D Array(array=w368, index=1) -> (first subarray=w365:dbl[])  [unwired: 1 out]
                    }
                    frame #2 {
                      n113 = local read "Number of Steps Left (must be even)"() -> (w384:dbl)
                      n114 = local read "loop iteration"() -> (w382:i32)
                      n115 = Divide(x=w384, y=2) -> (x/y=w383:dbl)
                      n116 = Equal?(x=w383, y=w382) -> (x = y?=w381:bool)
                      n117 = case shown="True" w381 {
                        tunnel: w390 -> [_ w397]
                        tunnel: w389 -> [w391 w393]
                        tunnel: [w392 w395] -> w388
                        tunnel: w387 -> [w392 w394]
                        tunnel: [w391 w393] -> w386
                        frame False {
                        }
                        frame True {
                          # "Use first\naxis only."
                          # "Wait until move\nhas stopped or\nstop is pressed"
                          # "Move first axis 0.01 mm\nrelative to its current\nposition."
                          n118 = Index Array(array=w397, index=2) -> (element=w402:string)
                          n119 = Build Array(w402) -> (w400:string[])
                          n120 = Absolute Value(x="Step Size (microns) Z") -> (abs(x)=w398:dbl[])
                          n121 = call "MVR.vi"("System no."=w393, "Axes to move"=w400, "Position values"=w398, "error in"=w394) -> ("error out"=w406:errorcluster)  [unwired: 1 in, 14 out]
                          n122 = call "General wait for movement to stop.vi"("System no."=w393, "Axes to wait for"=w400, "error in"=w406) -> ("error out"=w401:errorcluster)  [unwired: 5 in, 11 out]
                          n123 = call "POS?.vi"("System no."=w393, "Axes to query"=w400, "All axes?"=TRUE, "error in"=w401) -> ("Position"=→"Position 6":dbl[], "error out"=w405:errorcluster)  [unwired: 1 in, 13 out]
                          n124 = call "ERR?.vi"("System no."=w393, "error in"=w405) -> ("error out"=w404:errorcluster)  [unwired: 17 out]
                          n125 = call "GCSTranslateError.vi"("error in"=w404) -> ("error out"=w395:errorcluster)  [unwired: 18 out]
                        }
                      }
                    }
                  }
                  n126 = Build Array (concatenate)(w246, w237) -> (w245:dbl[][])
                  n127 = Array To Spreadsheet String(array=w245, 3:"%f" ("format string")) -> (spreadsheet string=w248:string)  [unwired: 1 in]
                }
                n128 = local read "Number of Steps Left (must be even)"() -> (w211:dbl)
                n129 = local read "Number of Steps Down"() -> (w218:dbl)
                n130 = call "File Dialog3"("start path"=path "C:/Users/Raman Lab/Desktop/Molly") -> ("selected path"=w226:path)  [unwired: 11 in, 3 out]
                n131 = local read "Exposure 2"() -> (w213:dbl)
                n132 = call <userlib>:"CameraShutter.vi"("Camera Handle"=w225, "error in"=w223) -> ("Camera Handle"=w224:u32, "error out"=w222:errorcluster)  [unwired: 3 in]
                n133 = Number To Fractional String(number=w218) -> (F-format string=w217:string)  [unwired: 3 in]
                n134 = Number To Decimal String(number=w211) -> (decimal integer string=w210:string)  [unwired: 1 in]
                n135 = Number To Decimal String(number=w213) -> (decimal integer string=w214:string)  [unwired: 1 in]
                n136 = Concatenate Strings(w217, "\r\n", w210, "\r\n", w214, "\r\n", w219) -> (w228:string)
                n137 = Write to Text File(file (use dialog)=w226, text=w228) -> ()  [unwired: 2 in, 3 out]
              }
              frame #3 {
                n138 = Tick Count (ms)() -> (millisecond timer value=w408:u32)
              }
            }
            n139 = Subtract(x=w178, y=w179) -> (x-y=→"Execution Time (ms)":u32)
          }
        }
      }
      frame "Stage Control" {
        n140 = case shown="True" "?" {
          tunnel: w409 -> [_ w451]
          tunnel: w410 -> [_ w450]
          frame False {
          }
          frame True {
            n141 = stacked-sequence {
              seq-local: [w453 _] -> [_ w473]
              seq-local: [w452 _] -> [_ w472]
              tunnel: w450 -> [w454 _]
              tunnel: w451 -> [w455 _]
              frame #0 {
                n142 = stacked-sequence {
                  tunnel: w455 -> [w459]
                  tunnel: w454 -> [w458]
                  tunnel: [w457] -> w452
                  tunnel: [w456] -> w453
                  frame #0 {
                    w471 = cluster{"S/N":string, "USB Search?":bool} {"S/N"="", "USB Search?"=TRUE}  # USB settings
                    w467 = u16 2 items=["RS232", "TCP/IP", "USB"] ("Interface")
                    w466 = cluster{"Portnumber":i32, "Baudrate":u16} {"Portnumber"=0, "Baudrate"=5}  # RS232 settings
                    w465 = T4 {"Host address/name"="", "Port"=50000, "Board"=0, "TCP/IP Search?"=TRUE}  # TCP/IP settings
                    # "TRUE: We want to\nmove the axis to its middle\nposition"
                    # "System number is one"
                    n143 = call "E727_Configuration_Setup.vi"("System no."=w458, "USB settings"=w471, "Are stages connected?"=bool[] [TRUE, TRUE, FALSE], "Change servo status to ON?"=TRUE ("Use dialog to define\nconnected stages?"), "Perform autozero?"=FALSE ("Use dialog to define\nconnected stages?"), "error in"=w459, "Interface"=w467, "RS232 settings"=w466, "TCP/IP settings"=w465, "Stop wave generator\noutput (if any)"=TRUE ("All axes?"), "Move to middle?"=FALSE) -> ("All conn. axes"=w456:string[], "error out"=w461:errorcluster)  [unwired: 3 in, 4 out]
                    n144 = call "POS?.vi"("System no."=w458, "Axes to query"=w456, "All axes?"=TRUE, "error in"=w461) -> ("Position"=→"Position 4":dbl[], "error out"=w457:errorcluster)  [unwired: 1 in, 13 out]
                  }
                }
              }
              frame #1 {
                n145 = stacked-sequence {
                  tunnel: w473 -> [w476]
                  tunnel: w472 -> [w475]
                  frame #0 {
                    w474 = 1
                    # "Use first\naxis only."
                    # "Wait until move\nhas stopped or\nstop is pressed"
                    # "Move first axis 0.01 mm\nrelative to its current\nposition."
                    n146 = local read "Step Size (microns) Y"() -> (w477:dbl[])
                    n147 = Index Array(array=w476, index=0) -> (element=w481:string)
                    n148 = Build Array(w481) -> (w479:string[])
                    n149 = call "MVR.vi"("System no."=w474, "Axes to move"=w479, "Position values"=w477, "error in"=w475) -> ("error out"=w485:errorcluster)  [unwired: 1 in, 14 out]
                    n150 = call "General wait for movement to stop.vi"("System no."=w474, "Axes to wait for"=w479, "error in"=w485) -> ("error out"=w480:errorcluster)  [unwired: 5 in, 11 out]
                    n151 = call "POS?.vi"("System no."=w474, "Axes to query"=w479, "All axes?"=TRUE, "error in"=w480) -> ("Position"=→"Position 5":dbl[], "error out"=w484:errorcluster)  [unwired: 1 in, 13 out]
                    n152 = call "ERR?.vi"("System no."=w474, "error in"=w484) -> ("error out"=w483:errorcluster)  [unwired: 17 out]
                    n153 = call "GCSTranslateError.vi"("error in"=w483) -> ()  [unwired: 19 out]
                  }
                }
              }
            }
          }
        }
        n154 = case shown="True" "?" {
          tunnel: w409 -> [_ w414]
          tunnel: w410 -> [_ w413]
          frame False {
          }
          frame True {
            n155 = stacked-sequence {
              seq-local: [w416 _] -> [_ w436]
              seq-local: [w415 _] -> [_ w435]
              tunnel: w413 -> [w417 _]
              tunnel: w414 -> [w418 _]
              frame #0 {
                n156 = stacked-sequence {
                  tunnel: w418 -> [w422]
                  tunnel: w417 -> [w421]
                  tunnel: [w420] -> w415
                  tunnel: [w419] -> w416
                  frame #0 {
                    w434 = cluster{"S/N":string, "USB Search?":bool} {"S/N"="", "USB Search?"=TRUE}  # USB settings
                    w430 = u16 2 items=["RS232", "TCP/IP", "USB"] ("Interface")
                    w429 = cluster{"Portnumber":i32, "Baudrate":u16} {"Portnumber"=0, "Baudrate"=5}  # RS232 settings
                    w428 = T4 {"Host address/name"="", "Port"=50000, "Board"=0, "TCP/IP Search?"=TRUE}  # TCP/IP settings
                    # "TRUE: We want to\nmove the axis to its middle\nposition"
                    # "System number is one"
                    n157 = call "E727_Configuration_Setup.vi"("System no."=w421, "USB settings"=w434, "Are stages connected?"=bool[] [TRUE, TRUE, FALSE], "Change servo status to ON?"=TRUE ("Use dialog to define\nconnected stages?"), "Perform autozero?"=FALSE ("Use dialog to define\nconnected stages?"), "error in"=w422, "Interface"=w430, "RS232 settings"=w429, "TCP/IP settings"=w428, "Stop wave generator\noutput (if any)"=TRUE ("All axes?"), "Move to middle?"=FALSE) -> ("All conn. axes"=w419:string[], "error out"=w424:errorcluster)  [unwired: 3 in, 4 out]
                    n158 = call "POS?.vi"("System no."=w421, "Axes to query"=w419, "All axes?"=TRUE, "error in"=w424) -> ("Position"=→"Position 7":dbl[], "error out"=w420:errorcluster)  [unwired: 1 in, 13 out]
                  }
                }
              }
              frame #1 {
                n159 = stacked-sequence {
                  tunnel: w436 -> [w439]
                  tunnel: w435 -> [w438]
                  frame #0 {
                    w437 = 1
                    # "Use first\naxis only."
                    # "Wait until move\nhas stopped or\nstop is pressed"
                    # "Move first axis 0.01 mm\nrelative to its current\nposition."
                    n160 = local read "Step Size (microns) X"() -> (w440:dbl[])
                    n161 = Index Array(array=w439, index=1) -> (element=w444:string)
                    n162 = Build Array(w444) -> (w442:string[])
                    n163 = call "MVR.vi"("System no."=w437, "Axes to move"=w442, "Position values"=w440, "error in"=w438) -> ("error out"=w448:errorcluster)  [unwired: 1 in, 14 out]
                    n164 = call "General wait for movement to stop.vi"("System no."=w437, "Axes to wait for"=w442, "error in"=w448) -> ("error out"=w443:errorcluster)  [unwired: 5 in, 11 out]
                    n165 = call "POS?.vi"("System no."=w437, "Axes to query"=w442, "All axes?"=TRUE, "error in"=w443) -> ("Position"=→"Position 8":dbl[], "error out"=w447:errorcluster)  [unwired: 1 in, 13 out]
                    n166 = call "ERR?.vi"("System no."=w437, "error in"=w447) -> ("error out"=w446:errorcluster)  [unwired: 17 out]
                    n167 = call "GCSTranslateError.vi"("error in"=w446) -> ()  [unwired: 19 out]
                  }
                }
              }
            }
          }
        }
      }
    }
    n168 = global read "GlobalCamOpen.vi" "Camera Opened"() -> (w25:u32)
    n169 = Not(x="Release Camera") -> (.not. x?=w17:bool)
    n170 = Greater Than 0?(x=w25) -> (x > 0?=w24:bool)
    n171 = And(x=w17, y=w24) -> (x .and. y?=→"Camera Opened":bool)
    n172 = Wait Until Next ms Multiple(millisecond multiple=5) -> ()  [unwired: 1 out]
  }
  n173 = call <userlib>:"CameraClose.vi"("error in"=w8, "Camera Handle"=w5) -> ("error out"=w7:errorcluster)
  n174 = call "Close connection if open.vi"("System no."=w1) -> ("error out"=→"error out 2":errorcluster)  [unwired: 2 in, 16 out]
  n175 = call <userlib>:"UninitToolkit.vi"("error in"=w7) -> ("error out"=→"error out":errorcluster)
